vi "Call Import With Path.vi"(8 "error in (no error)":errorcluster, 10 "Path":path, 11 "Node Ptr":u64) -> (0 "error out":errorcluster, 3 "Node Ptr out":u64)   [LabVIEW 2017, in "NI-SWITCH Import Export Unit Tests.lvclass"]
uses:
  NI-SWITCH Import Export Unit Tests.lvclass
  System Explorer/Import Configuration RTM.vi
  System Explorer/NI-SWITCH System Explorer.lvlib
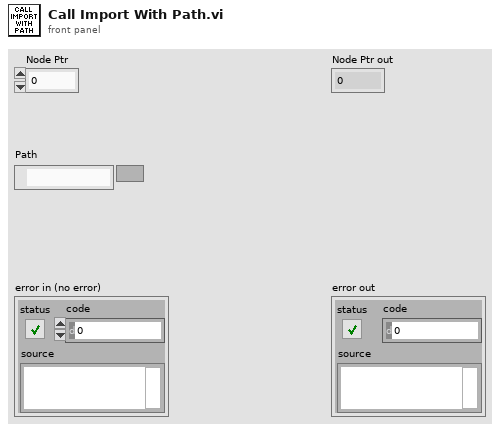
[diagram p1: front panel]
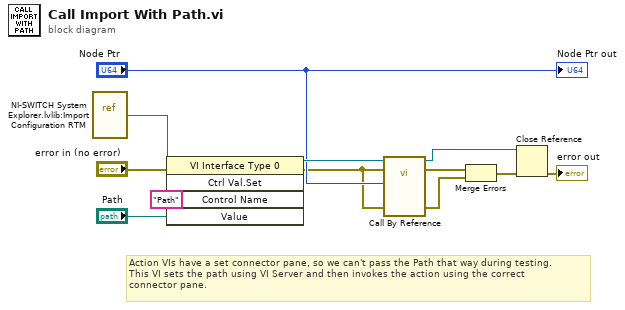
[diagram p0: block diagram]
diagram:
  # "Action VIs have a set connector pane, so we can't pass the Path that way during testing.\nThis VI sets the path using VI Server and then invokes the action using the correct\nconnector pane."
  n1 = vi-ref "NI-SWITCH System Explorer.lvlib:Import Configuration RTM.vi"() -> (w1:refnum<vi>)
  n2 = invoke class="VI Interface Type 0" method="Ctrl Val.Set"(reference=w1, error in="error in (no error)", "Control Name"="Path", "Value"="Path") -> (reference out=w11:refnum<vi>, error out=w7:errorcluster)  [unwired: 1 in, 3 out]
  n3 = call-by-ref "?"(reference=w11, error in=w7, 8:"error in (no error)"=w7, "Node Ptr"="Node Ptr") -> (reference out=w3:refnum<vi>, error out=w6:errorcluster, 0:"error out"=w5:errorcluster)  [unwired: 9 in]
  n4 = Merge Errors(w6, w5) -> (w4:errorcluster)
  n5 = Close Reference(reference=w3, error in (no error)=w4) -> (error out=→"error out":errorcluster)
  "Node Ptr out" <- "Node Ptr"
